vi "PH_Sequencer.SCR Start Slow Devices.vi"(0 "i ref in":refnum<vi>, 5 "error in (no error)":errorcluster) -> (14 "i ref out":refnum<vi>, 19 "error out":errorcluster)   [LabVIEW 2014, in "PH_Sequencer.lvlib"]
doc: "This VI sends a state change request to the Seq SM. If the sequencer is in state \"Stand by\", and \"Ready to Shot\" = true, \"Start Slow Devices\" is requested."
uses:
  PH_Sequencer.lvlib
  CSCore/BaseSM/BaseSM.lvlib
  PH_Common/PH_Common.lvlib
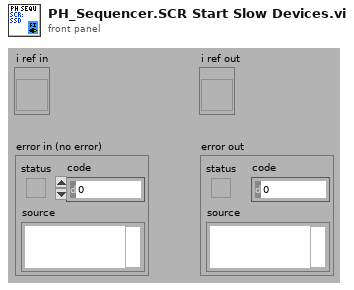
[diagram p1: front panel]
types:
  T1 = typedef "PH_Sequencer.lvlib/PH_Sequencer.i attribute.ctl" = cluster{"GUI Refs":cluster{"Main Off":refnum<vi>, "Fire":refnum<vi>, "Status":refnum<vi>, "Ready":refnum<vi>, "Waiting Time":refnum<vi>, "Timeout":refnum<vi>, "PPMA Ready":refnum<vi>, "Sequencer SM State":refnum<vi>, "PPPA Ready":refnum<vi>, "Calorimeter":refnum<vi>, "Beamline Ready":refnum<vi>, "Clear Beamline":refnum<vi>, "Linkage PPMA Rods":refnum<vi>, "Linkage Current PA":refnum<vi>, "Linkage Current MA":refnum<vi>, "Timing Ready":refnum<vi>, "State Timing":refnum<vi>, "Force Timing":refnum<vi>, "PSDB Shot Comment":refnum<vi>, "State PA Backreflection":refnum<vi>, "Beamline Z6 Ready":refnum<vi>, "Clear Z6 Beamline":refnum<vi>, "Sequence length":refnum<vi>, "Timing Mode":refnum<vi>, "Slow Trigger Settings":refnum<vi>, "Experiment Description":refnum<vi>, "State PSDB":refnum<vi>, "PSDB Ready":refnum<vi>, "Set PSDB Settings":refnum<vi>, "Get PSDB Info":refnum<vi>, "Take Snapshot":refnum<vi>, "Shottype":refnum<vi>, "Experiment":refnum<vi>, "Phase Frontends":refnum<vi>, "PP 45mm PILC in use":refnum<vi>}, "Status Info":cluster{"Machine Status":T2, "WaitingTime":i32, "Timeout":bool}, "Readyness":cluster{"Ready to shot":bool, "PPMA Ready":bool, "PPPA Ready":bool, "BL Ready":bool, "Timing Ready":bool, "BL Z6 Ready":bool, "PSDBReady":bool}, "Instancenames":cluster{"PPMA Rods":string, "PP Current Meas":string, "PH Beamline Chief":string, "PA Backrefl Meas":string, "Z6 Beamline Chief":string}, "Data to read":bool, "Calorimeter":cluster{"Instancename":string, "On":bool, "linked":bool}, "Linkage":cluster{"PPMA Rods":bool, "PP Current Meas":bool, "PHELIX Beamline Chief":bool, "PA Backrefl Meas":bool, "Z6 Beamline Chief":bool}, "Timing":cluster{"Instance":string, "linked":bool, "Status":T2, "Timing Mode":T3, "Slow Trigger Settings":T4, "Info available":cluster{"ext SlowTrigger":bool, "T2":bool, "Mode":bool, "Delay Slow Trigger":bool, "Phase FEs":bool}, "FE Phase":T5}, "Service ID R2S":i32, "PSDB":cluster{"Controller Instance":string, "Controller Status":T2, "Controller linked":bool, "Settings acknowledged":bool, "Current Experiment ID":i16, "Current Shot Type":i16, "Current Comment":string, "Remember Settings":bool, "Write 2 early":bool}, "PSDB Data":cluster{"Main Off?":bool, "Sequence Length":dbl, "Sequence startet":timestamp}, "6P 4Q Positions":cluster{"Instancename":string, "linked":bool, "Position":T6}[], "PUs":T7[]}
  T2 = typedef "PH_StatusHandler.lvlib/PH_StatusHandler.Status.ctl" = i16
  T3 = typedef "PH_Timing.lvlib/PH_Timing.Timing Mode.ctl" = cluster{"T2":i16, "Modeselector":enum32{"10 Hz", "0.5 Hz", "Shot"}}
  T4 = typedef "PH_Timing.lvlib/PH_Timing.Slow Trigger Settings.ctl" = cluster{"Delay":dbl, "externally triggered?":bool}
  T5 = typedef "PH_Timing.lvlib/PH_Timing.Phase FEs.ctl" = cluster{"Phase":dbl}
  T6 = typedef "PH_4_Pos_Selector.lvlib/PH_4_Pos_Selector.Position Selector.ctl" = u16
  T7 = typedef "PH_Sequencer.lvlib/PH_Sequencer.Head.ctl" = cluster{"PowerUnit":T8, "GUI Ref":refnum<vi>, "Information":T9, "linked?":bool, "GUI Ref Current Voltage":refnum<vi>}
  T8 = typedef "PH_PP_Common.lvlib/PH_PP_Common.PUs.ctl" = enum16{"no Info", "PA-19mm-1", "PA-19mm-2", "PA-45mm-PILC", "PA-45mm-MAIN", "MA-PU-1", "MA-PU-2", "MA-PU-3", "MA-PU-4", "MA-PU-5", "MA-PU-6", "MA-FR", "MA-PILC", "PA-45mm-DP"}
  T9 = typedef "PH_Sequencer.lvlib/PH_Sequencer.PU Information.ctl" = cluster{"State":T2, "Waiting Time [s]":dbl, "PU State SM":T10, "PU Timeout SM":T10}
  T10 = typedef "PH_PowerUnit_BaseClass.lvlib/PH_PowerUnit_BaseClass.SM States.ctl" = enum16{".", "Stand by", "Switch PU on", "Configure", "Set Default Voltage", "Set STANDBY", "Set READY", "Wait for Shot Cmd", "Open Dump Rods", "Open Ross Relais", "Close Ross Relais", "Switch PSU on", "Switch PSU off", "Charge", "Switch GD Channel on", "Close Dump Rods", "Rods-TO", "RR-TO", "PSU-TO", "Trigger-TO"}
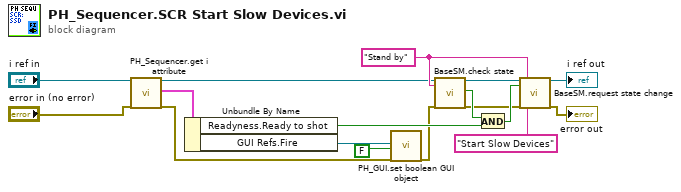
[diagram p0: block diagram]
diagram:
  w17 = "Stand by" ("requested state")
  n1 = call "PH_Sequencer.get i attribute.vi"("i ref in"="i ref in", "error in (no error)"="error in (no error)") -> ("i ref out"=w6:refnum<vi>, "i attribute"=w9:T1, "error out"=w3:errorcluster)  [unwired: 15 in]
  n2 = Unbundle By Name(w9) -> ("Readyness.Ready to shot"=w14:bool, "GUI Refs.Fire"=w4:refnum<vi>)
  n3 = call "PH_GUI.set boolean GUI object.vi"("Boolean Knob GUI Ref"=w4, "Value"=FALSE, "error in (no error)"=w3) -> ("error out"=w1:errorcluster)  [unwired: 16 in]
  n4 = call "BaseSM.check state.vi"("i ref in"=w6, "requestedState"=w17, "error in (no error)"=w1) -> ("i ref out"=w10:refnum<vi>, "OK"=w13:bool, "error out"=w11:errorcluster)  [unwired: 11 in, 3 out]
  n5 = And(x=w13, y=w14) -> (x .and. y?=w15:bool)
  n6 = call "BaseSM.request state change.vi"("i ref in"=w10, "change"=w15, "error in (no error)"=w11, "allowed current state"=w17, "requested state"="Start Slow Devices" ("next state")) -> ("i ref out"=→"i ref out":refnum<vi>, "error out"=→"error out":errorcluster)  [unwired: 11 in, 2 out]
